vi "Check Unified Actor.vi"(10 "Unified Actor":refnum<class "Actor.lvclass">) -> (2 "Error":errorcluster)   [LabVIEW 2020, in "jettl.lvlib"]
uses:
  jettl.lvlib
  Actor/Actor.lvclass
  Lifetime.ctl
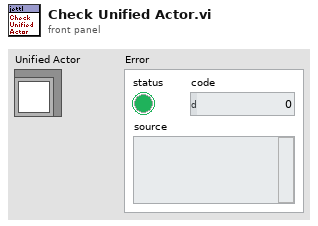
[diagram p1: front panel]
types:
  T1 = typedef "jettl.lvlib/Lifetime.ctl" = enum16{"Init", "Spawn", "Setup", "Teardown Before Running", "Running", "Stop Called", "Stopping With Children", "Stopping Without Children", "Teardown After Running", "Stopped"}
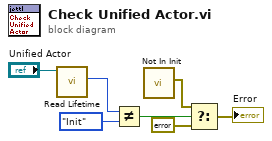
[diagram p0: block diagram]
diagram:
  n1 = call-dynamic "Read Lifetime.vi"("Actor in"="Unified Actor") -> ("Lifetime"=w1:T1)  [unwired: 10 in]
  n2 = Not Equal?(x=w1, y=Lifetime."Init") -> (x != y?=w4:bool)
  n3 = call "Not In Init.vi"() -> ("Error"=w7:errorcluster)  [unwired: 11 in]
  n4 = Select(t=w7, s=w4, f=errorcluster {"status"=FALSE, "code"=0, "source"=""}) -> (s? t:f=→"Error":errorcluster)
